vi "Pause.vi"(8 "error in":errorcluster, 11 "4-20mA Settings In":T1={"Input DAQ Task"="", "Output DAQ Task"="", "Pressure Setpoint"=0.02, "Working?"=FALSE} {"Pressure Setpoint" min=0.004 max=0.02}) -> (0 "error out":errorcluster, 3 "4-20mA Settings Out":T1={"Input DAQ Task"="", "Output DAQ Task"="", "Pressure Setpoint"=0.02, "Working?"=FALSE} {"Pressure Setpoint" min=0.004 max=0.02})   [LabVIEW 2018]
uses:
  Pressure Regulator Module/Pressure Regulator/Controls/Pressure Regulator Module Device Settings.ctl
  Pressure Regulator Module/Pressure Regulator/Pressure Regulator Module.lvlib
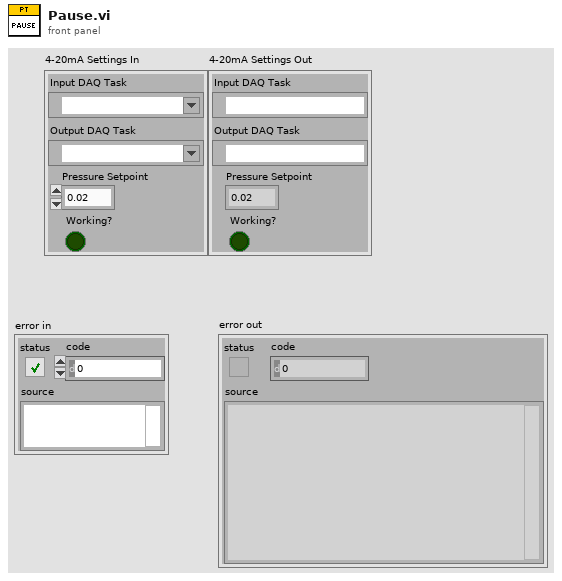
[diagram p1: front panel]
types:
  T1 = typedef "Pressure Regulator Module.lvlib/Pressure Regulator Module Device Settings.ctl" = cluster{"Input DAQ Task":refnum<k21>, "Output DAQ Task":refnum<k21>, "Pressure Setpoint":dbl, "Working?":bool}
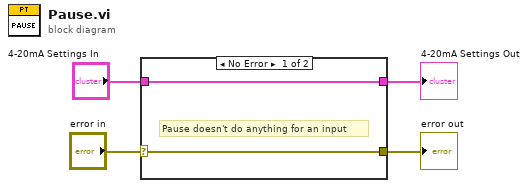
[diagram p0: block diagram]
diagram:
  n1 = case shown="No Error" "error in" {
    selector: "error in" -> [w5 w8]
    tunnel: "4-20mA Settings In" -> [w6 w7]
    tunnel: [w5 w8] -> w3
    tunnel: [w6 w7] -> w1
    frame No Error {
      # "Pause doesn't do anything for an input"
    }
    frame Error {
    }
  }
  "error out" <- w3
  "4-20mA Settings Out" <- w1
